vi "散斑物体作用.vi"(9 "图像1024一维数组":dbl[](array[numeric]), 10 "数值输入":dbl, 11 "光源数组":dbl[][](array[numeric])) -> (3 "数值输出":dbl)   [LabVIEW 2018]
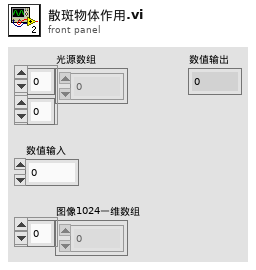
[diagram p1: front panel]
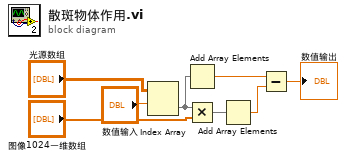
[diagram p0: block diagram]
diagram:
  n1 = Index Array(array="光源数组", index (row)="数值输入") -> (element=w3:dbl[])  [unwired: 1 in]
  n2 = Add Array Elements(numeric array=w3) -> (sum=w5:dbl)
  n3 = Multiply(x=w3, y="图像1024一维数组") -> (x*y=w2:dbl[])
  n4 = Add Array Elements(numeric array=w2) -> (sum=w4:dbl)
  n5 = Subtract(x=w5, y=w4) -> (x-y=→"数值输出":dbl)
